vi "ComputerName.vi"(8 "error in (no error)":errorcluster) -> (0 "error out":errorcluster, 5 "String/Binary data":string)   [LabVIEW 2013]
uses:
  <vilib>/registry/registry.llb/Registry RtKey.ctl
  <vilib>/registry/registry.llb/Read Registry Value Simple STR.vi
panel:
  in  "value":string="ComputerName"
  in  "root key (HKEY_LOCAL_MACHINE)":T1=enum."HKEY_LOCAL_MACHINE"
  in  "subkey":string="System\\CurrentControlSet\\Control\\ComputerName\\ComputerName"
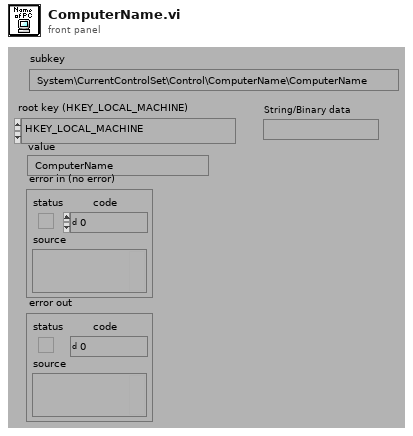
[diagram p1: front panel]
types:
  T1 = typedef "Registry RtKey.ctl" = enum32{"HKEY_CLASSES_ROOT", "HKEY_CURRENT_USER", "HKEY_LOCAL_MACHINE", "HKEY_USERS", "HKEY_PERFORMANCE_DATA", "HKEY_CURRENT_CONFIG", "HKEY_DYN_DATA"}
  T2 = typedef "Registry refnum.ctl" = refnum<k1>
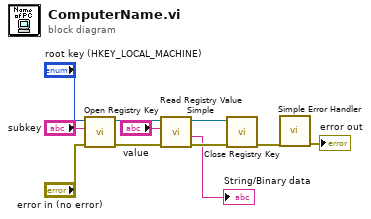
[diagram p0: block diagram]
diagram:
  n1 = call <vilib>:"Open Registry Key.vi"("error in (no error)"="error in (no error)", "subkey"="subkey", "root key (HKEY_LOCAL_MACHINE)"="root key (HKEY_LOCAL_MACHINE)") -> ("error out"=w11:errorcluster, "refnum out"=w10:T2)  [unwired: 7 in]
  n2 = call-poly <vilib>:"Read Registry Value Simple.vi"("error in (no error)"=w11, "value"="value", "refnum"=w10) -> ("error out"=w9:errorcluster, "String/Binary data"=→"String/Binary data":string, "refnum out"=w8:T2)  [unwired: 3 in, 1 out]
  n3 = call <vilib>:"Close Registry Key.vi"("error in (no error)"=w9, "refnum"=w8) -> ("error out"=w7:errorcluster)  [unwired: 5 in]
  n4 = call <vilib>:"Simple Error Handler.vi"("error in (no error)"=w7) -> ("error out"=→"error out":errorcluster)  [unwired: 4 in, 4 out]
